vi "TestCode2.vi"() -> ()   [LabVIEW 2012]
uses:
  <userlib>/rosforlv/Gazebo/AxesDrawing/ReferenceFrame.ctl
panel:
  in  "Angle (degrees) 2":dbl(slide)=-44.081632653061234 scale=-180.0..180.0
  in  "Angle (degrees)":dbl(slide) scale=-180.0..180.0
  out "3D Picture":refnum<vi>(3d-picture)
  out "Final 2 Frame":T1={"nx"=1.0, "ny"=0.0, "nz"=0.0, "nw"=0.0, "ox"=0.0, "oy"=1.0, "oz"=0.0, "ow"=0.0, "ax"=0.0, "ay"=0.0, "az"=1.0, "aw"=0.0, "Px"=0.2, "Py"=0.0, "Pz"=0.5, "Pw"=1.0} {"Pw" format="%.2f"; "Pz" format="%.2f"; "Py" format="%.2f"; "Px" format="%.2f"; "aw" format="%.2f"; "az" format="%.2f"; "ay" format="%.2f"; "ax" format="%.2f"; "ow" format="%.2f"; "nw" format="%.2f"; "oz" format="%.2f"; "oy" format="%.2f"; "ox" format="%.2f"; "nz" format="%.2f"; "ny" format="%.2f"; "nx" format="%.2f"}
  out "Final Frame":T1={"nx"=0.7183493500977276, "ny"=-0.6956825506034864, "nz"=0.0, "nw"=0.0, "ox"=0.6956825506034864, "oy"=0.7183493500977276, "oz"=0.0, "ow"=0.0, "ax"=0.0, "ay"=0.0, "az"=1.0, "aw"=0.0, "Px"=0.2, "Py"=0.0, "Pz"=0.5, "Pw"=1.0} {"Pw" format="%.2f"; "Pz" format="%.2f"; "Py" format="%.2f"; "Px" format="%.2f"; "aw" format="%.2f"; "az" format="%.2f"; "ay" format="%.2f"; "ax" format="%.2f"; "ow" format="%.2f"; "nw" format="%.2f"; "oz" format="%.2f"; "oy" format="%.2f"; "ox" format="%.2f"; "nz" format="%.2f"; "ny" format="%.2f"; "nx" format="%.2f"}
  in  "World Frame":T1={"nx"=1.0, "ny"=0.0, "nz"=0.0, "nw"=0.0, "ox"=0.0, "oy"=1.0, "oz"=0.0, "ow"=0.0, "ax"=0.0, "ay"=0.0, "az"=1.0, "aw"=0.0, "Px"=0.3, "Py"=0.1, "Pz"=0.2, "Pw"=1.0} {"Pw" format="%.2f"; "Pz" format="%.2f"; "Py" format="%.2f"; "Px" format="%.2f"; "aw" format="%.2f"; "az" format="%.2f"; "ay" format="%.2f"; "ax" format="%.2f"; "ow" format="%.2f"; "nw" format="%.2f"; "oz" format="%.2f"; "oy" format="%.2f"; "ox" format="%.2f"; "nz" format="%.2f"; "ny" format="%.2f"; "nx" format="%.2f"}
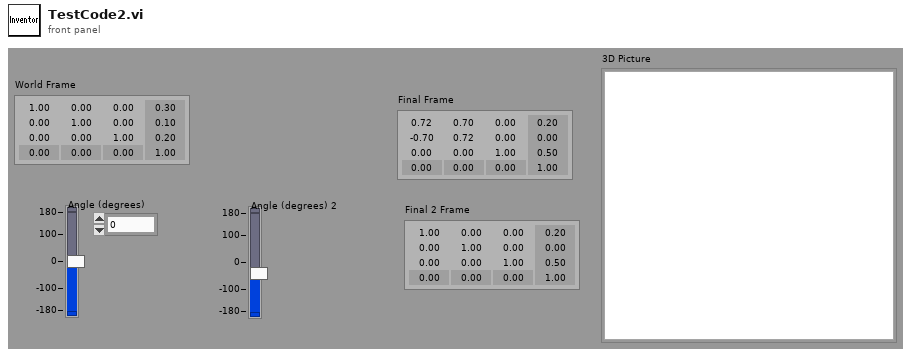
[diagram p1: front panel]
types:
  T1 = typedef "ReferenceFrame.ctl" = cluster{"nx":dbl, "ny":dbl, "nz":dbl, "nw":dbl, "ox":dbl, "oy":dbl, "oz":dbl, "ow":dbl, "ax":dbl, "ay":dbl, "az":dbl, "aw":dbl, "Px":dbl, "Py":dbl, "Pz":dbl, "Pw":dbl}
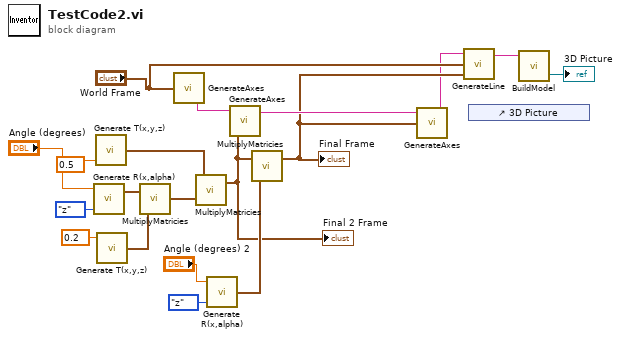
[diagram p0: block diagram]
diagram:
  n1 = call <userlib>:"Generate R(x,alpha).vi"("Axis"=enum16{"x", "y", "z"}."z", "Angle (degrees)"="Angle (degrees)") -> ("Final Frame"=w11:T1)  [unwired: 1 in]
  n2 = call <userlib>:"Generate T(x,y,z).vi"("Z"=0.5 ("X")) -> ("Final Frame"=w9:T1)  [unwired: 2 in]
  n3 = call <userlib>:"Generate T(x,y,z).vi"("X"=0.2) -> ("Final Frame"=w10:T1)  [unwired: 2 in]
  n4 = call <userlib>:"MultiplyMatricies.vi"("B"=w10, "A"=w11) -> ("AxB"=w8:T1)  [unwired: 1 out]
  n5 = call <userlib>:"GenerateAxes.vi"("Frame"="World Frame") -> ("Text Out"=w13:string)  [unwired: 5 in]
  n6 = call <userlib>:"MultiplyMatricies.vi"("B"=w8, "A"=w9) -> ("AxB"=w6:T1)  [unwired: 1 out]
  "Final 2 Frame" <- w6
  n7 = call <userlib>:"Generate R(x,alpha).vi"("Axis"=enum16{"x", "y", "z"}."z", "Angle (degrees)"="Angle (degrees) 2") -> ("Final Frame"=w7:T1)  [unwired: 1 in]
  n8 = call <userlib>:"GenerateAxes.vi"("Text In"=w13, "Frame"=w6) -> ("Text Out"=w12:string)  [unwired: 4 in]
  n9 = call <userlib>:"MultiplyMatricies.vi"("B"=w7, "A"=w6) -> ("AxB"=w5:T1)  [unwired: 1 out]
  "Final Frame" <- w5
  n10 = call <userlib>:"GenerateAxes.vi"("Text In"=w12, "Frame"=w5) -> ("Text Out"=w3:string)  [unwired: 4 in]
  n11 = call <userlib>:"GenerateLine.vi"("Frame End"=w5, "Frame Start"="World Frame", "Text In"=w3) -> ("Text Out"=w2:string)  [unwired: 1 in]
  n12 = control-ref of="3D Picture"() -> ()  [unwired: 1 out]
  n13 = call <userlib>:"BuildModel.vi"("urdf in"=w2) -> ("3D Picture"=→"3D Picture":refnum<vi>)  [unwired: 3 in, 1 out]
